vi "Convert CAL String to timestamp.vi"(10 "abbreviated date string":string) -> (2 "time stamp":timestamp)   [LabVIEW 2011]
uses:
  <vilib>/Utility/miscctls.llb/LVDateTimeRec.ctl
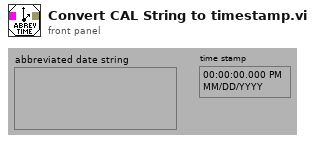
[diagram p1: front panel]
types:
  T1 = typedef "LVDateTimeRec.ctl" = cluster{"fractional second":dbl, "second":i32, "minute":i32, "hour":i32, "day of month":i32, "month":i32, "year":i32, "day of week":i32, "day of year":i32, "DST":i32}
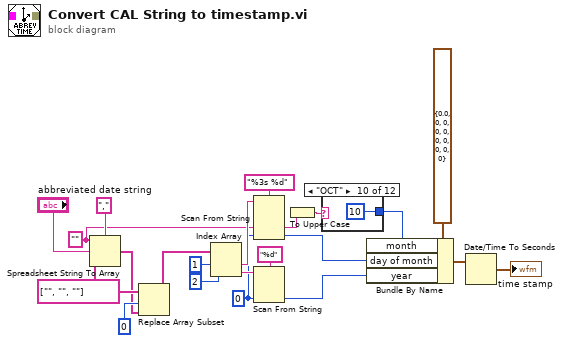
[diagram p0: block diagram]
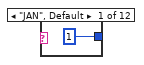
[diagram p2: hidden frame]
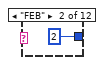
[diagram p3: hidden frame]
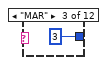
[diagram p4: hidden frame]
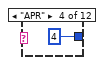
[diagram p5: hidden frame]
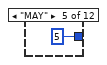
[diagram p6: hidden frame]
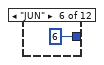
[diagram p7: hidden frame]
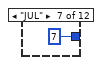
[diagram p8: hidden frame]
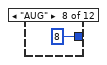
[diagram p9: hidden frame]
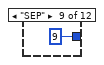
[diagram p10: hidden frame]
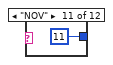
[diagram p11: hidden frame]
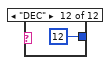
[diagram p12: hidden frame]
diagram:
  w6 = 0 ("default value 1")
  w5 = "" ("abbreviated date string")
  w4 = string[] ["", "", ""] ("array type (2D Dbl)")
  n1 = Spreadsheet String To Array(delimiter (Tab)=",", format string=w5, spreadsheet string="abbreviated date string", array type (2D Dbl)=w4) -> (array=w2:string[])
  n2 = Replace Array Subset(array=w4, new element=w2, index=0) -> (w1:string[])
  n3 = Index Array(array=w1, index #1=1 ("index"), index #2=2 ("index")) -> (element #1=w19:string, element #2=w16:string)
  n4 = Scan From String(format string="%3s %d", input string=w19, default 1=w5, default 2=w6) -> (output 1=w7:string, output 2=w13:i32)  [unwired: 2 in, 3 out]
  n5 = Scan From String(format string="%d", input string=w16, default 1=w6) -> (output 1=w12:i32)  [unwired: 2 in, 3 out]
  n6 = To Upper Case(1:w7) -> (0:w8:string)
  n7 = case shown="\"OCT\"" w8 {
    tunnel: [1 2 3 4 5 6 7 8 9 10 11 12] -> w14
    frame "JAN", Default {
    }
    frame "FEB" {
    }
    frame "MAR" {
    }
    frame "APR" {
    }
    frame "MAY" {
    }
    frame "JUN" {
    }
    frame "JUL" {
    }
    frame "AUG" {
    }
    frame "SEP" {
    }
    frame "OCT" {
    }
    frame "NOV" {
    }
    frame "DEC" {
    }
  }
  n8 = Bundle By Name(cluster=T1 {"fractional second"=0.0, "second"=0, "minute"=0, "hour"=0, "day of month"=0, "month"=0, "year"=0, "day of week"=0, "day of year"=0, "DST"=0} ("date time rec"), "month"=w14, "day of month"=w13, "year"=w12) -> (w11:T1)
  n9 = Date/Time To Seconds(2:w11) -> (0:→"time stamp":timestamp)  [unwired: 1 out]
